vi "UnpackFrame.vi"(8 "error in":errorcluster caption="错误输入（无错误）", 9 "FramePara":T1, 10 "原指令码":string, 11 "StrIn":string) -> (0 "error out":errorcluster caption="错误输出", 2 "data":string, 3 "反馈结果":bool)   [LabVIEW 2013]
panel:
  out "校验码":bool
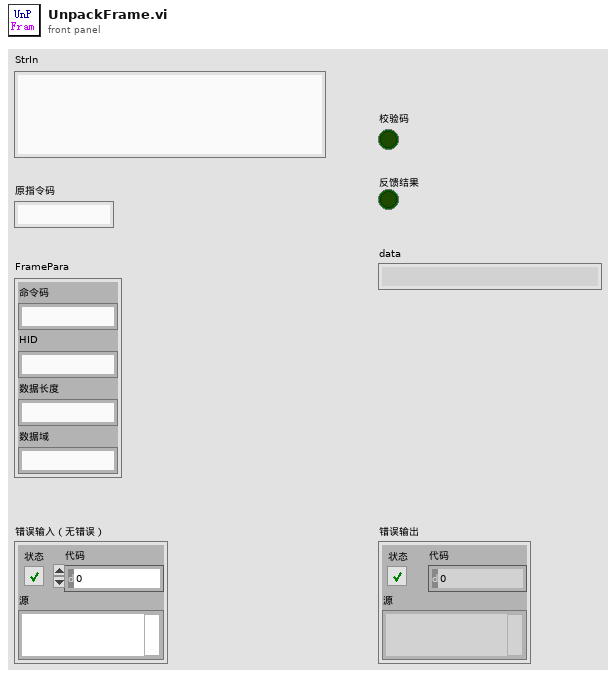
[diagram p1: front panel]
types:
  T1 = cluster{"命令码":string, "HID":string, "数据长度":string, "数据域":string}
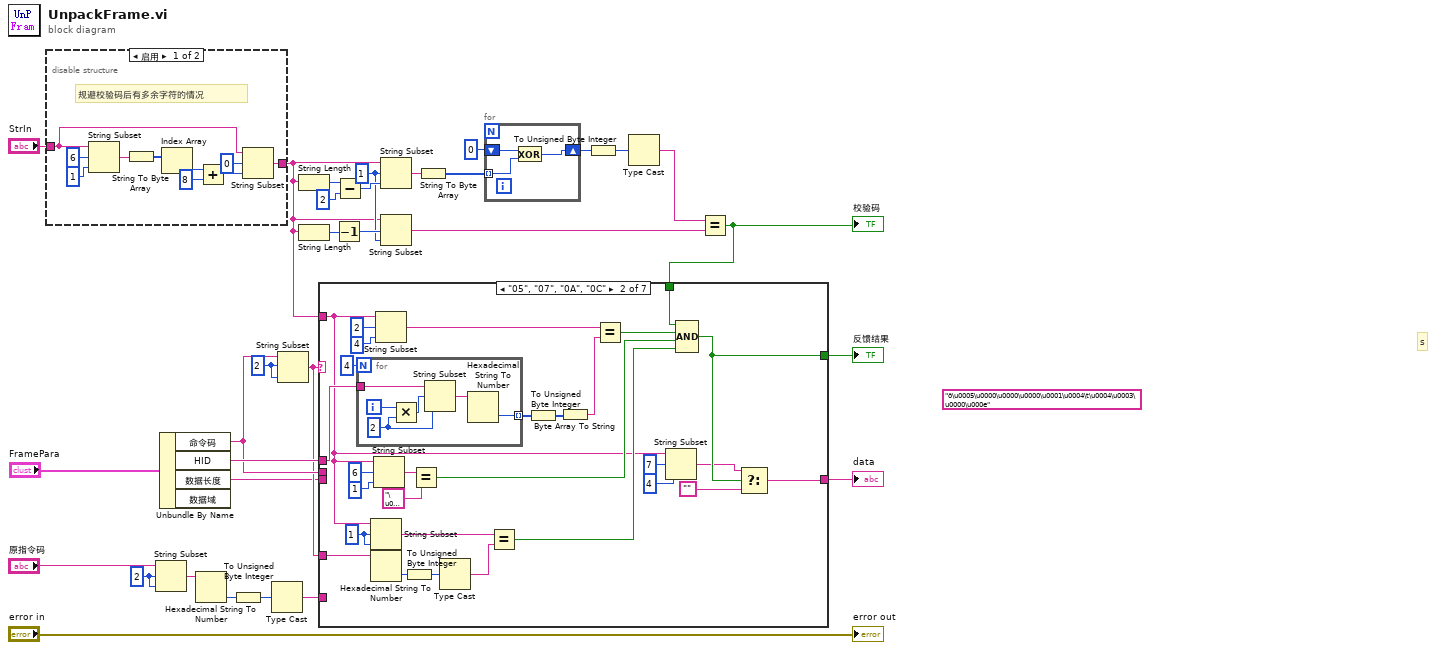
[diagram p0: block diagram]
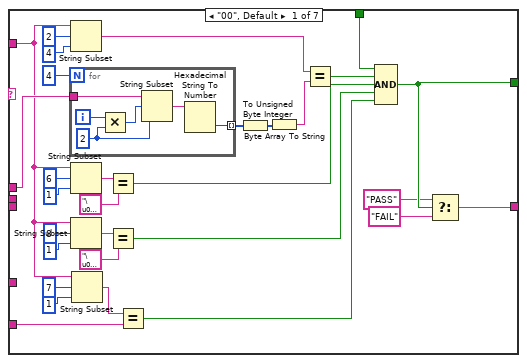
[diagram p3: hidden frame]
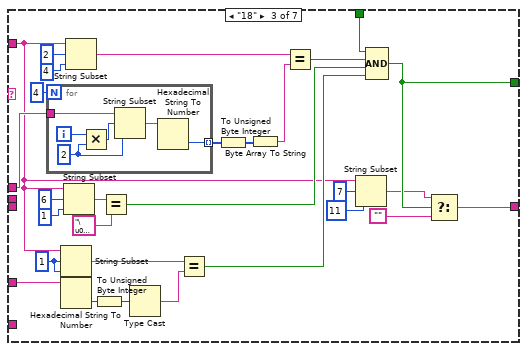
[diagram p4: hidden frame]
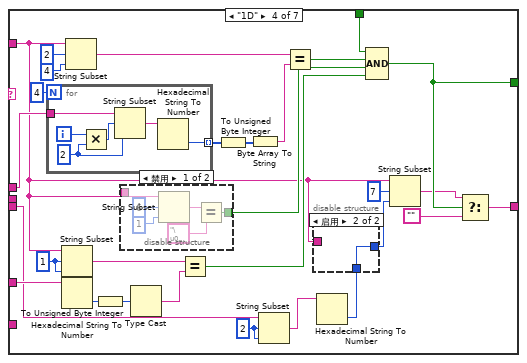
[diagram p5: hidden frame]
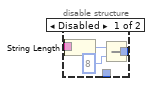
[diagram p6: hidden frame]
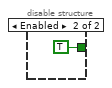
[diagram p7: hidden frame]
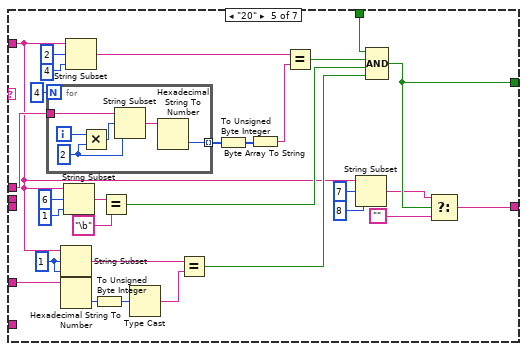
[diagram p8: hidden frame]
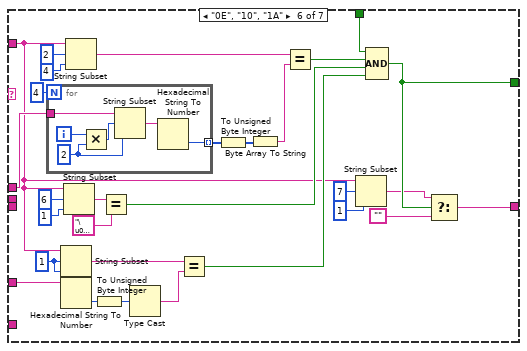
[diagram p9: hidden frame]
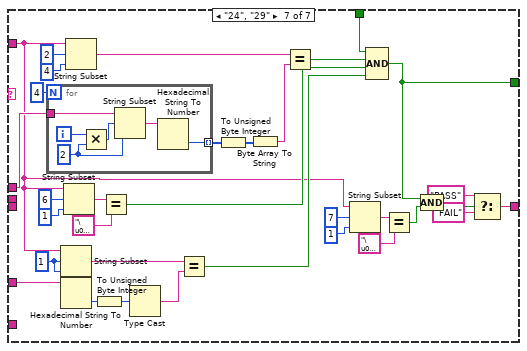
[diagram p10: hidden frame]
diagram:
  (unwired) "ð\u0005\u0000\u0000\u0000\u0001\u0004\t\u0004\u0003\u0000\u000e" ("响应")
  w9 = 2 ("偏移量(0)")
  w16 = 2
  w20 = 1 ("偏移量(0)")
  # "s"
  n1 = disable-structure shown="启用" {
    disable-tunnel: "StrIn" -> [w33 _]
    disable-tunnel: [w32 _] -> w2
    frame Enabled {
      # "规避校验码后有多余字符的情况"
      n2 = String Subset(string=w33, offset (0)=6 ("长度（剩余）"), length (rest)=1 ("长度（剩余）")) -> (substring=w39:string)
      n3 = String To Byte Array(string=w39) -> (unsigned byte array=w38:u8[])
      n4 = Index Array(array=w38) -> (element=w37:u8)  [unwired: 1 in]
      n5 = Add(x=w37, y=u8 8) -> (x+y=w35:u8)
      n6 = String Subset(string=w33, offset (0)=0 ("偏移量(0)"), length (rest)=w35) -> (substring=w32:string)
    }
    frame Disabled {
    }
  }
  n7 = String Subset(string="原指令码", offset (0)=w9, length (rest)=w9) -> (substring=w8:string)
  n8 = Unbundle By Name("FramePara") -> ("命令码"=w12:string, "HID"=w17:string, "数据长度"=w1:string)  [unwired: 1 out]
  n9 = Hexadecimal String To Number(string=w8) -> (number=w6:u32)  [unwired: 2 in, 1 out]
  n10 = To Unsigned Byte Integer(number=w6) -> (unsigned 8bit integer=w7:u8)
  n11 = Type Cast(x=w7) -> (*(type *) &x=w5:string)  [unwired: 1 in]
  n12 = String Subset(string=w12, offset (0)=w16, length (rest)=w16) -> (substring=w4:string)
  n13 = String Length(string=w2) -> (length=w30:i32)
  n14 = String Length(string=w2) -> (length=w22:i32)
  n15 = Decrement(x=w22) -> (x-1=w21:i32)
  n16 = Subtract(x=w30, y=2) -> (x-y=w28:i32)
  n17 = String Subset(string=w2, offset (0)=w20, length (rest)=w28) -> (substring=w27:string)
  n18 = String Subset(string=w2, offset (0)=w21, length (rest)=w20) -> (substring=w18:string)
  n19 = String To Byte Array(string=w27) -> (unsigned byte array=w25:u8[])
  n20 = for {
    shift-right: [w42] -> w24
    shift-left: u8 0 -> [w44]
    tunnel: w25 -> [w43] mode=indexing
    n21 = Exclusive Or(1:w43, 2:w44) -> (0:w42:u8)
  }
  n22 = To Unsigned Byte Integer(number=w24) -> (unsigned 8bit integer=w23:u8)
  n23 = Type Cast(x=w23) -> (*(type *) &x=w19:string)  [unwired: 1 in]
  n24 = Equal?(x=w19, y=w18) -> (x = y?=w15:bool)
  "校验码" <- w15
  n25 = case shown="\"05\", \"07\", \"0A\", \"0C\"" w4 {
    tunnel: w2 -> [w49 w86 w121 w156 w203 w238 w272]
    tunnel: w17 -> [w52 w101 w136 w171 w218 w253 w292]
    tunnel: w15 -> [w63 w106 w141 w176 w223 w258 w297]
    tunnel: [w59 w87 w122 w161 w204 w239 w278] -> w14
    tunnel: [w56 w82 w117 w158 w199 w234 w271] -> w13
    tunnel: w12 -> [_ _ _ _ _ _ _]
    tunnel: w4 -> [_ w93 w128 w167 w210 w245 w284]
    tunnel: w5 -> [w46 _ _ _ _ _ _]
    tunnel: w1 -> [_ _ _ w154 _ _ _]
    frame "00", Default {
      n26 = for {
        N: 4 -> [_]
        tunnel: w52 -> [w78]
        tunnel: [w75] -> w54 mode=indexing
        i -> [w80]
        w77 = 2
        n27 = Multiply(x=w80, y=w77) -> (x*y=w79:i32)
        n28 = String Subset(string=w78, offset (0)=w79, length (rest)=w77) -> (substring=w76:string)
        n29 = Hexadecimal String To Number(string=w76) -> (number=w75:u32)  [unwired: 2 in, 1 out]
      }
      n30 = String Subset(string=w49, offset (0)=2, length (rest)=4) -> (substring=w72:string)
      n31 = String Subset(string=w49, offset (0)=6, length (rest)=1) -> (substring=w64:string)
      n32 = String Subset(string=w49, offset (0)=8, length (rest)=1) -> (substring=w67:string)
      n33 = String Subset(string=w49, offset (0)=7, length (rest)=1) -> (substring=w47:string)
      n34 = Equal?(x=w64, y="\u0002") -> (x = y?=w61:bool)
      n35 = Equal?(x=w67, y="\u0001") -> (x = y?=w60:bool)
      n36 = Equal?(x=w47, y=w46) -> (x = y?=w45:bool)
      n37 = To Unsigned Byte Integer(number=w54) -> (unsigned 8bit integer=w55:u8[])
      n38 = Byte Array To String(unsigned byte array=w55) -> (string=w51:string)
      n39 = Equal?(x=w72, y=w51) -> (x = y?=w62:bool)
      n40 = Compound Arithmetic op=AND(w63, w62, w61, w60, w45) -> (w59:bool)
      n41 = Select(t="PASS", s=w59, f="FAIL") -> (s? t:f=w56:string)
    }
    frame "05", "07", "0A", "0C" {
      w94 = 1
      n42 = for {
        N: 4 -> [_]
        tunnel: w101 -> [w113]
        tunnel: [w110] -> w103 mode=indexing
        i -> [w115]
        w112 = 2
        n43 = Multiply(x=w115, y=w112) -> (x*y=w114:i32)
        n44 = String Subset(string=w113, offset (0)=w114, length (rest)=w112) -> (substring=w111:string)
        n45 = Hexadecimal String To Number(string=w111) -> (number=w110:u32)  [unwired: 2 in, 1 out]
      }
      n46 = String Subset(string=w86, offset (0)=w94, length (rest)=w94) -> (substring=w90:string)
      n47 = Hexadecimal String To Number(string=w93) -> (number=w92:u32)  [unwired: 2 in, 1 out]
      n48 = String Subset(string=w86, offset (0)=6, length (rest)=1) -> (substring=w96:string)
      n49 = String Subset(string=w86, offset (0)=2, length (rest)=4) -> (substring=w107:string)
      n50 = To Unsigned Byte Integer(number=w92) -> (unsigned 8bit integer=w91:u8)
      n51 = Equal?(x=w96, y="\u0004") -> (x = y?=w95:bool)
      n52 = Type Cast(x=w91) -> (*(type *) &x=w89:string)  [unwired: 1 in]
      n53 = Equal?(x=w90, y=w89) -> (x = y?=w88:bool)
      n54 = To Unsigned Byte Integer(number=w103) -> (unsigned 8bit integer=w104:u8[])
      n55 = Byte Array To String(unsigned byte array=w104) -> (string=w100:string)
      n56 = Equal?(x=w107, y=w100) -> (x = y?=w105:bool)
      n57 = String Subset(string=w86, offset (0)=7 ("偏移量(0)"), length (rest)=4 ("长度（剩余）")) -> (substring=w85:string)
      n58 = Compound Arithmetic op=AND(w106, w105, w95, w88) -> (w87:bool)
      n59 = Select(t=w85, s=w87, f="") -> (s? t:f=w82:string)
    }
    frame "18" {
      w129 = 1
      n60 = for {
        N: 4 -> [_]
        tunnel: w136 -> [w148]
        tunnel: [w145] -> w138 mode=indexing
        i -> [w150]
        w147 = 2
        n61 = Multiply(x=w150, y=w147) -> (x*y=w149:i32)
        n62 = String Subset(string=w148, offset (0)=w149, length (rest)=w147) -> (substring=w146:string)
        n63 = Hexadecimal String To Number(string=w146) -> (number=w145:u32)  [unwired: 2 in, 1 out]
      }
      n64 = String Subset(string=w121, offset (0)=w129, length (rest)=w129) -> (substring=w125:string)
      n65 = Hexadecimal String To Number(string=w128) -> (number=w127:u32)  [unwired: 2 in, 1 out]
      n66 = String Subset(string=w121, offset (0)=6, length (rest)=1) -> (substring=w131:string)
      n67 = String Subset(string=w121, offset (0)=2, length (rest)=4) -> (substring=w142:string)
      n68 = To Unsigned Byte Integer(number=w127) -> (unsigned 8bit integer=w126:u8)
      n69 = Equal?(x=w131, y="\u000b") -> (x = y?=w130:bool)
      n70 = Type Cast(x=w126) -> (*(type *) &x=w124:string)  [unwired: 1 in]
      n71 = Equal?(x=w125, y=w124) -> (x = y?=w123:bool)
      n72 = To Unsigned Byte Integer(number=w138) -> (unsigned 8bit integer=w139:u8[])
      n73 = Byte Array To String(unsigned byte array=w139) -> (string=w135:string)
      n74 = Equal?(x=w142, y=w135) -> (x = y?=w140:bool)
      n75 = String Subset(string=w121, offset (0)=7 ("偏移量(0)"), length (rest)=11 ("长度（剩余）")) -> (substring=w120:string)
      n76 = Compound Arithmetic op=AND(w141, w140, w130, w123) -> (w122:bool)
      n77 = Select(t=w120, s=w122, f="") -> (s? t:f=w117:string)
    }
    frame "1D" {
      w153 = 2 ("偏移量(0)")
      w168 = 1
      n78 = for {
        N: 4 -> [_]
        tunnel: w171 -> [w195]
        tunnel: [w192] -> w173 mode=indexing
        i -> [w197]
        w194 = 2
        n79 = Multiply(x=w197, y=w194) -> (x*y=w196:i32)
        n80 = String Subset(string=w195, offset (0)=w196, length (rest)=w194) -> (substring=w193:string)
        n81 = Hexadecimal String To Number(string=w193) -> (number=w192:u32)  [unwired: 2 in, 1 out]
      }
      n82 = String Subset(string=w156, offset (0)=w168, length (rest)=w168) -> (substring=w164:string)
      n83 = Hexadecimal String To Number(string=w167) -> (number=w166:u32)  [unwired: 2 in, 1 out]
      n84 = String Subset(string=w156, offset (0)=2, length (rest)=4) -> (substring=w177:string)
      n85 = To Unsigned Byte Integer(number=w166) -> (unsigned 8bit integer=w165:u8)
      n86 = disable-structure shown="禁用" {
        disable-tunnel: [w186 TRUE] -> w169
        disable-tunnel: w156 -> [w185 _]
        frame Disabled {
          n87 = String Subset(string=w185, offset (0)=6, length (rest)=1) -> (substring=w187:string)
          n88 = Equal?(x=w187, y="\u0019") -> (x = y?=w186:bool)
        }
        frame Enabled {
        }
      }
      n89 = Type Cast(x=w165) -> (*(type *) &x=w163:string)  [unwired: 1 in]
      n90 = Equal?(x=w164, y=w163) -> (x = y?=w162:bool)
      n91 = To Unsigned Byte Integer(number=w173) -> (unsigned 8bit integer=w174:u8[])
      n92 = Byte Array To String(unsigned byte array=w174) -> (string=w170:string)
      n93 = String Subset(string=w154, offset (0)=w153, length (rest)=w153) -> (substring=w152:string)
      n94 = Equal?(x=w177, y=w170) -> (x = y?=w175:bool)
      n95 = Hexadecimal String To Number(string=w152) -> (number=w151:u32)  [unwired: 2 in, 1 out]
      n96 = disable-structure shown="启用" {
        disable-tunnel: w156 -> [w183 _]
        disable-tunnel: [w180 w184] -> w155
        disable-tunnel: w151 -> [_ w184]
        frame Disabled {
          n97 = String Length(string=w183) -> (length=w182:i32)
          n98 = Subtract(x=w182, y=8 ("长度（剩余）")) -> (x-y=w180:i32)
        }
        frame Enabled {
        }
      }
      n99 = Compound Arithmetic op=AND(w176, w175, w169, w162) -> (w161:bool)
      n100 = String Subset(string=w156, offset (0)=7 ("偏移量(0)"), length (rest)=w155) -> (substring=w160:string)
      n101 = Select(t=w160, s=w161, f="") -> (s? t:f=w158:string)
    }
    frame "20" {
      w211 = 1
      n102 = for {
        N: 4 -> [_]
        tunnel: w218 -> [w230]
        tunnel: [w227] -> w220 mode=indexing
        i -> [w232]
        w229 = 2
        n103 = Multiply(x=w232, y=w229) -> (x*y=w231:i32)
        n104 = String Subset(string=w230, offset (0)=w231, length (rest)=w229) -> (substring=w228:string)
        n105 = Hexadecimal String To Number(string=w228) -> (number=w227:u32)  [unwired: 2 in, 1 out]
      }
      n106 = String Subset(string=w203, offset (0)=w211, length (rest)=w211) -> (substring=w207:string)
      n107 = Hexadecimal String To Number(string=w210) -> (number=w209:u32)  [unwired: 2 in, 1 out]
      n108 = String Subset(string=w203, offset (0)=6, length (rest)=1) -> (substring=w213:string)
      n109 = String Subset(string=w203, offset (0)=2, length (rest)=4) -> (substring=w224:string)
      n110 = To Unsigned Byte Integer(number=w209) -> (unsigned 8bit integer=w208:u8)
      n111 = Equal?(x=w213, y="\b") -> (x = y?=w212:bool)
      n112 = Type Cast(x=w208) -> (*(type *) &x=w206:string)  [unwired: 1 in]
      n113 = Equal?(x=w207, y=w206) -> (x = y?=w205:bool)
      n114 = To Unsigned Byte Integer(number=w220) -> (unsigned 8bit integer=w221:u8[])
      n115 = Byte Array To String(unsigned byte array=w221) -> (string=w217:string)
      n116 = Equal?(x=w224, y=w217) -> (x = y?=w222:bool)
      n117 = String Subset(string=w203, offset (0)=7 ("偏移量(0)"), length (rest)=8 ("长度（剩余）")) -> (substring=w202:string)
      n118 = Compound Arithmetic op=AND(w223, w222, w212, w205) -> (w204:bool)
      n119 = Select(t=w202, s=w204, f="") -> (s? t:f=w199:string)
    }
    frame "0E", "10", "1A" {
      w246 = 1
      n120 = for {
        N: 4 -> [_]
        tunnel: w253 -> [w265]
        tunnel: [w262] -> w255 mode=indexing
        i -> [w267]
        w264 = 2
        n121 = Multiply(x=w267, y=w264) -> (x*y=w266:i32)
        n122 = String Subset(string=w265, offset (0)=w266, length (rest)=w264) -> (substring=w263:string)
        n123 = Hexadecimal String To Number(string=w263) -> (number=w262:u32)  [unwired: 2 in, 1 out]
      }
      n124 = String Subset(string=w238, offset (0)=w246, length (rest)=w246) -> (substring=w242:string)
      n125 = Hexadecimal String To Number(string=w245) -> (number=w244:u32)  [unwired: 2 in, 1 out]
      n126 = String Subset(string=w238, offset (0)=6, length (rest)=1) -> (substring=w248:string)
      n127 = String Subset(string=w238, offset (0)=2, length (rest)=4) -> (substring=w259:string)
      n128 = To Unsigned Byte Integer(number=w244) -> (unsigned 8bit integer=w243:u8)
      n129 = Equal?(x=w248, y="\u0001") -> (x = y?=w247:bool)
      n130 = Type Cast(x=w243) -> (*(type *) &x=w241:string)  [unwired: 1 in]
      n131 = Equal?(x=w242, y=w241) -> (x = y?=w240:bool)
      n132 = To Unsigned Byte Integer(number=w255) -> (unsigned 8bit integer=w256:u8[])
      n133 = Byte Array To String(unsigned byte array=w256) -> (string=w252:string)
      n134 = Equal?(x=w259, y=w252) -> (x = y?=w257:bool)
      n135 = String Subset(string=w238, offset (0)=7 ("偏移量(0)"), length (rest)=1 ("长度（剩余）")) -> (substring=w237:string)
      n136 = Compound Arithmetic op=AND(w258, w257, w247, w240) -> (w239:bool)
      n137 = Select(t=w237, s=w239, f="") -> (s? t:f=w234:string)
    }
    frame "24", "29" {
      w285 = 1
      n138 = for {
        N: 4 -> [_]
        tunnel: w292 -> [w304]
        tunnel: [w301] -> w294 mode=indexing
        i -> [w306]
        w303 = 2
        n139 = Multiply(x=w306, y=w303) -> (x*y=w305:i32)
        n140 = String Subset(string=w304, offset (0)=w305, length (rest)=w303) -> (substring=w302:string)
        n141 = Hexadecimal String To Number(string=w302) -> (number=w301:u32)  [unwired: 2 in, 1 out]
      }
      n142 = String Subset(string=w272, offset (0)=w285, length (rest)=w285) -> (substring=w281:string)
      n143 = Hexadecimal String To Number(string=w284) -> (number=w283:u32)  [unwired: 2 in, 1 out]
      n144 = String Subset(string=w272, offset (0)=6, length (rest)=1) -> (substring=w287:string)
      n145 = String Subset(string=w272, offset (0)=2, length (rest)=4) -> (substring=w298:string)
      n146 = To Unsigned Byte Integer(number=w283) -> (unsigned 8bit integer=w282:u8)
      n147 = Equal?(x=w287, y="\u0001") -> (x = y?=w286:bool)
      n148 = Type Cast(x=w282) -> (*(type *) &x=w280:string)  [unwired: 1 in]
      n149 = Equal?(x=w281, y=w280) -> (x = y?=w279:bool)
      n150 = To Unsigned Byte Integer(number=w294) -> (unsigned 8bit integer=w295:u8[])
      n151 = Byte Array To String(unsigned byte array=w295) -> (string=w291:string)
      n152 = Equal?(x=w298, y=w291) -> (x = y?=w296:bool)
      n153 = String Subset(string=w272, offset (0)=7, length (rest)=1) -> (substring=w277:string)
      n154 = Compound Arithmetic op=AND(w297, w296, w286, w279) -> (w278:bool)
      n155 = Equal?(x=w277, y="\u0001") -> (x = y?=w273:bool)
      n156 = Compound Arithmetic op=AND(w278, w273) -> (w270:bool)
      n157 = Select(t="PASS", s=w270, f="FAIL") -> (s? t:f=w271:string)
    }
  }
  "反馈结果" <- w14
  "data" <- w13
  "error out" <- "error in"
